vi "WriteResFile.vi"(4 "EMGstd":dbl[][](array[numeric]), 6 "EMGmean":dbl[][](array[numeric]), 8 "error in (no error)":errorcluster, 9 "Original File Name":string, 10 "Folder Path":path, 11 "EMG in":refnum<class "EMG.lvclass">) -> (0 "error out":errorcluster, 3 "EMG out":refnum<class "EMG.lvclass">)   [LabVIEW 2015, in "EMG.lvclass"]
uses:
  EMG.lvclass
  EMG.lvclass/EMG.ctl
  <vilib>/Utility/file.llb/Write To Spreadsheet File (string).vi
  <vilib>/Utility/file.llb/Write To Spreadsheet File (DBL).vi
  CustomVIs/CustomVI.lvlib
panel:
  out "EMGstd":dbl[][](array[numeric])
  out "Muscles":string[](array[string])
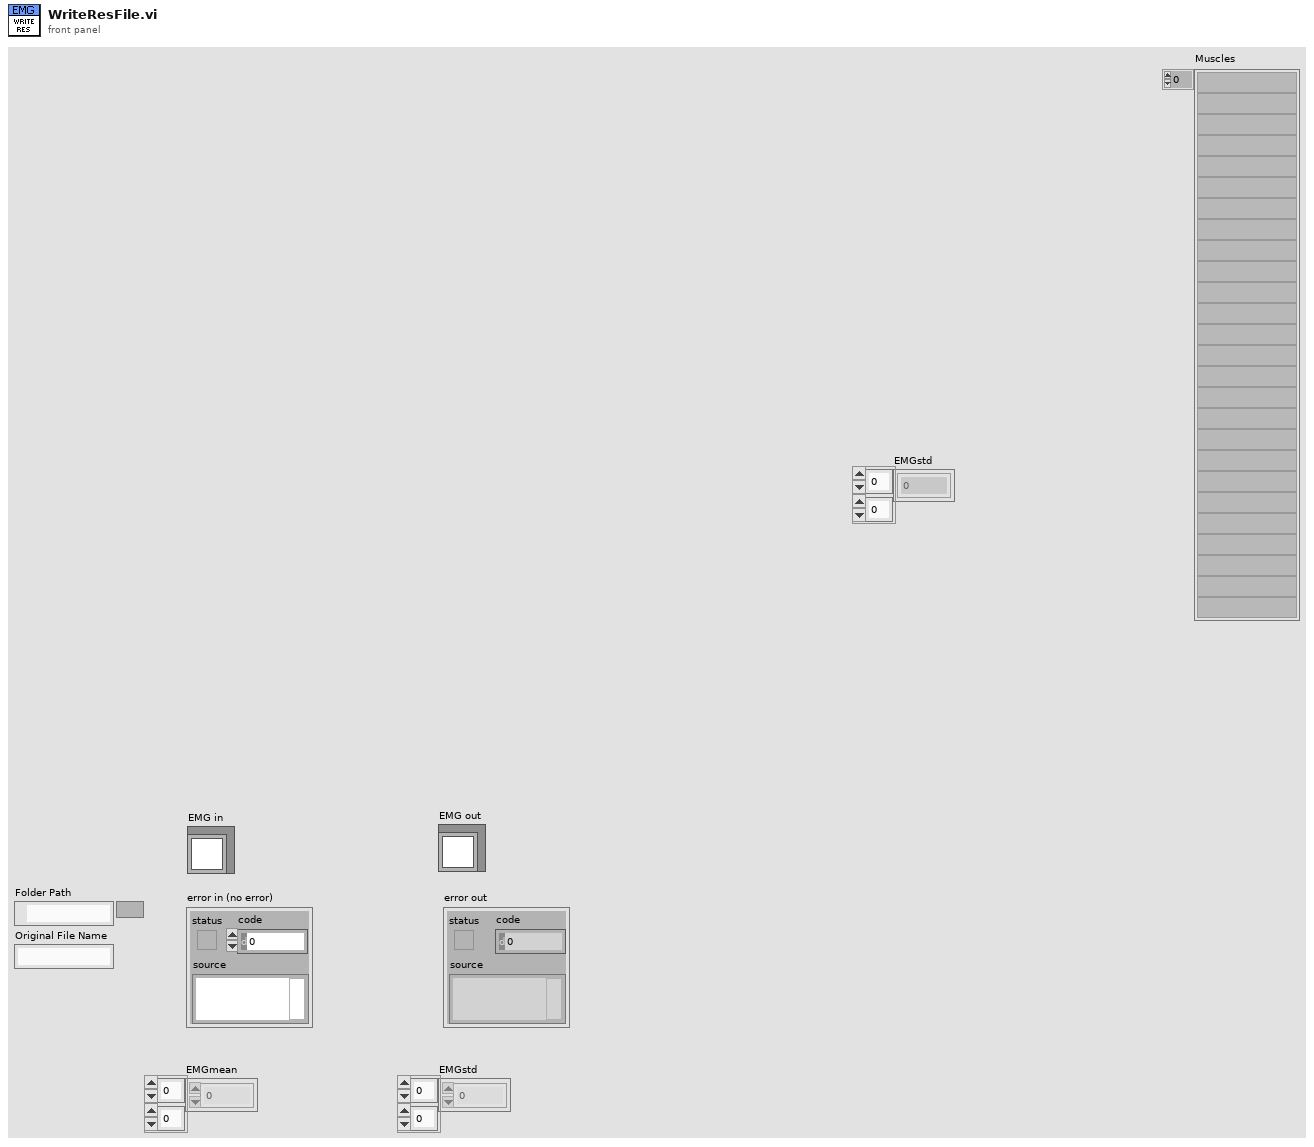
[diagram p1: front panel]
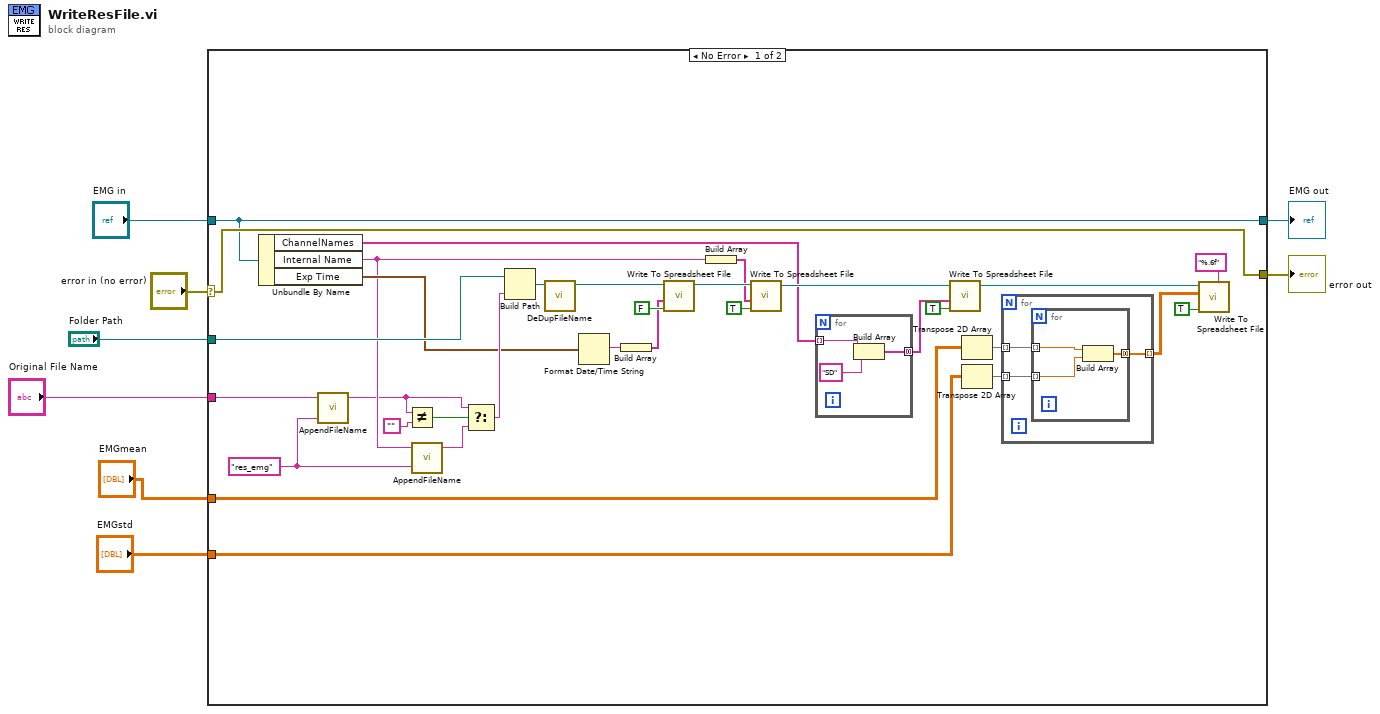
[diagram p0: block diagram]
diagram:
  n1 = case shown="No Error" "error in (no error)" {
    selector: "error in (no error)" -> [w15 w52]
    tunnel: [w15 w52] -> w8
    tunnel: "EMG in" -> [w14 w51]
    tunnel: [w14 w51] -> w5
    tunnel: "EMGmean" -> [w32 _]
    tunnel: "EMGstd" -> [w31 _]
    tunnel: "Folder Path" -> [w30 _]
    tunnel: "Original File Name" -> [w11 _]
    frame No Error {
      w9 = "res_emg" ("string")
      n2 = local read "EMGstd"() -> (w41:dbl[][])
      n3 = Transpose 2D Array(2D array=w41) -> ()  [unwired: 1 out]
      n4 = Unbundle By Name(w14) -> ("ChannelNames"=w17:string[], "Internal Name"=w13:string, "Exp Time"=w16:timestamp)
      n5 = call "AppendFileName.vi"("Appendix"=w9, "Filename"=w11) -> ("New Filename"=w10:string)  [unwired: 3 in]
      n6 = Not Equal?(x=w10, y="") -> (x != y?=w29:bool)
      n7 = call "AppendFileName.vi"("Appendix"=w9, "Filename"=w13) -> ("New Filename"=w12:string)  [unwired: 3 in]
      n8 = Select(t=w10, s=w29, f=w12) -> (s? t:f=w28:string)
      n9 = Build Path(base path=w30, name or relative path=w28) -> (appended path=w27:path)
      n10 = call "DeDupFileName.vi"("Path"=w27) -> ("Out Path"=w25:path)  [unwired: 8 in, 2 out]
      n11 = Format Date/Time String(seconds (now)=w16) -> (date/time string=w19:string)  [unwired: 2 in]
      n12 = Build Array(w19) -> (w18:string[])
      n13 = call-poly <vilib>:"Write To Spreadsheet File.vi"("append to file? (new file:F)"=FALSE, "1D data"=w18, "file path (dialog if empty)"=w25) -> ("new file path (Not A Path if cancelled)"=w22:path)  [unwired: 5 in]
      n14 = Build Array(w13) -> (w20:string[])
      n15 = call-poly <vilib>:"Write To Spreadsheet File.vi"("append to file? (new file:F)"=TRUE, "1D data"=w20, "file path (dialog if empty)"=w22) -> ("new file path (Not A Path if cancelled)"=w21:path)  [unwired: 5 in]
      n16 = for {
        tunnel: w17 -> [w44] mode=indexing
        tunnel: [w42] -> w33 mode=concatenating
        n17 = Build Array(w44, "SD") -> (w42:string[])
      }
      n18 = call-poly <vilib>:"Write To Spreadsheet File.vi"("append to file? (new file:F)"=TRUE, "1D data"=w33, "file path (dialog if empty)"=w21) -> ("new file path (Not A Path if cancelled)"=w38:path)  [unwired: 5 in]
      n19 = Transpose 2D Array(2D array=w32) -> (transposed array=w35:dbl[][])
      n20 = Transpose 2D Array(2D array=w31) -> (transposed array=w36:dbl[][])
      n21 = for {
        tunnel: w36 -> [w46] mode=indexing
        tunnel: w35 -> [w47] mode=indexing
        tunnel: [w45] -> w34 mode=indexing
        n22 = for {
          tunnel: w47 -> [w50] mode=indexing
          tunnel: w46 -> [w49] mode=indexing
          tunnel: [w48] -> w45 mode=concatenating
          n23 = Build Array(w50, w49) -> (w48:dbl[])
        }
      }
      n24 = call-poly <vilib>:"Write To Spreadsheet File.vi"("format (%.3f)"="%.6f", "append to file? (new file:F)"=TRUE, "2D data"=w34, "file path (dialog if empty)"=w38) -> ()  [unwired: 4 in, 1 out]
    }
    frame Error {
    }
  }
  "error out" <- w8
  "EMG out" <- w5
